vi "ArmTest_LE_and_XZ.vi"() -> ()   [LabVIEW 2020]
uses:
  <vilib>/Rock Robotics/WPI/ThirdParty/JAS_Junk/TrajLib/Trajectory_Library.lvlib
panel:
  out "Passed":bool
  out "Extend 2":dbl
  out "Lift 2":dbl
  out "z":dbl
  out "x":dbl
  in  "Lift":dbl
  in  "Extend":dbl
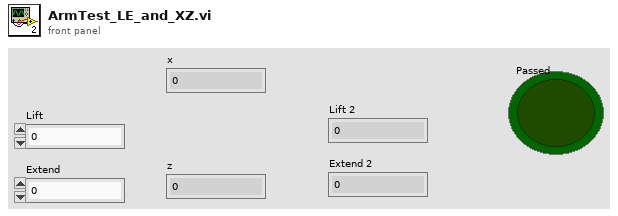
[diagram p1: front panel]
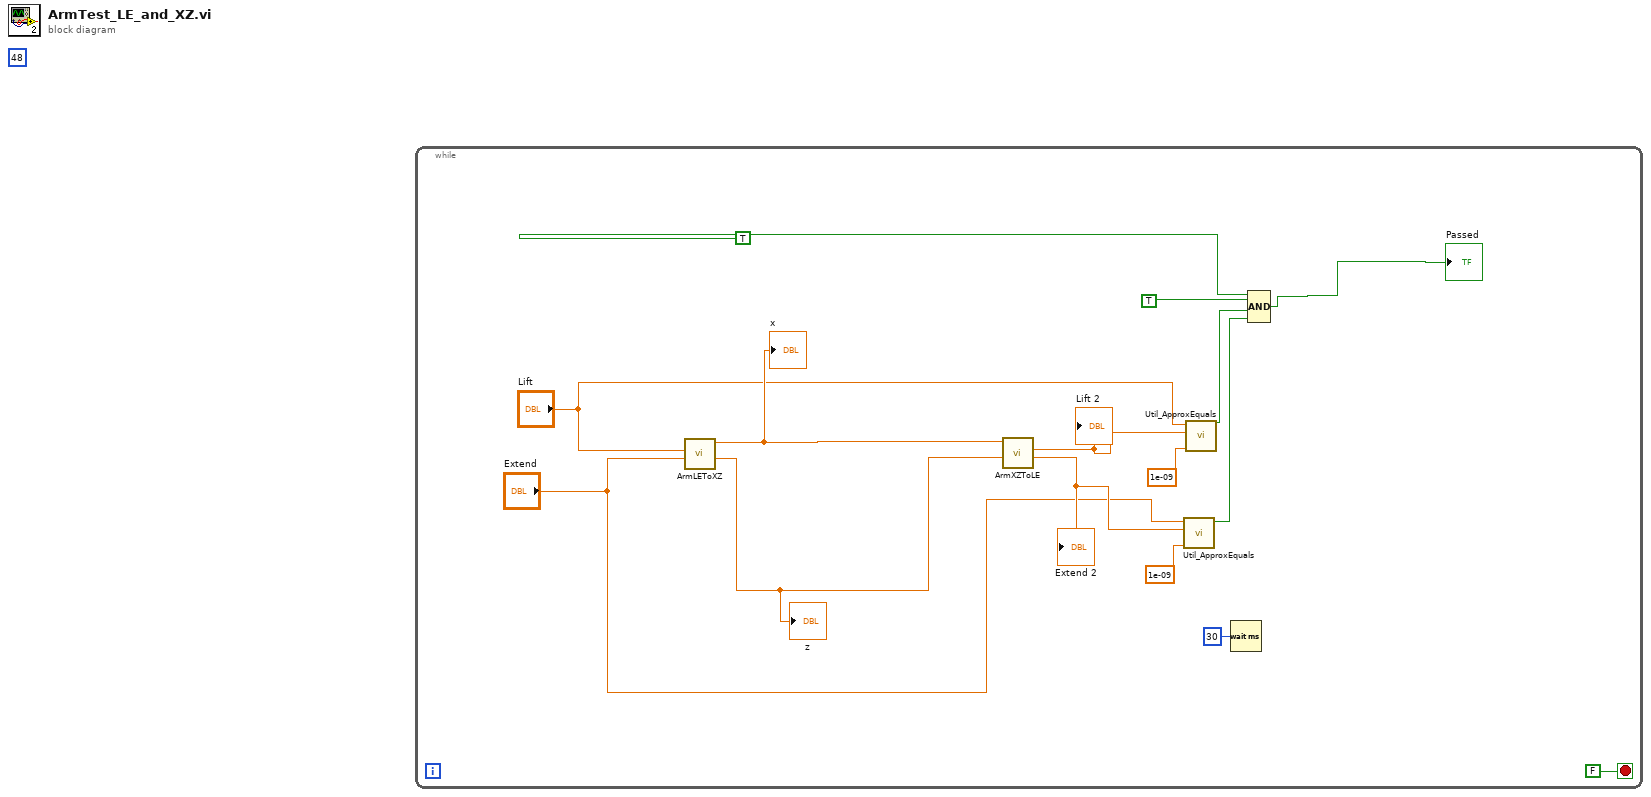
[diagram p0: block diagram]
diagram:
  (unwired) 48
  n1 = while {
    stop <- FALSE stop-if-true
    n2 = call "ArmLEToXZ.vi"("Extend"="Extend", "Lift"="Lift") -> ("z"=w12:dbl, "x"=w13:dbl)  [unwired: 8 in]
    "x" <- w13
    "z" <- w12
    n3 = call "ArmXZToLE.vi"("Z"=w12, "X"=w13) -> ("Extend"=w8:dbl, "Lift"=w9:dbl)  [unwired: 8 in]
    "Lift 2" <- w9
    "Extend 2" <- w8
    n4 = call <vilib>:"Util_ApproxEquals.vi"("Tolerance"=1e-09, "Value 2"=w8, "Value 1"="Extend") -> ("ApproxEquals"=w6:bool)  [unwired: 8 in]
    n5 = call <vilib>:"Util_ApproxEquals.vi"("Tolerance"=1e-09, "Value 2"=w9, "Value 1"="Lift") -> ("ApproxEquals"=w7:bool)  [unwired: 8 in]
    n6 = Wait (ms)(milliseconds to wait=u32 30) -> ()  [unwired: 1 out]
    n7 = Compound Arithmetic op=AND(TRUE, TRUE ("value"), w7, w6) -> (→"Passed":bool)
  }
